vi "FF_WriteAnkleTraj.vi"(8 "error in (no error)":errorcluster, 10 "AnkleTraj":T1(array[cluster]), 11 "ForceField in":refnum<class "ForceField.lvclass">) -> (0 "error out":errorcluster, 3 "ForceField out":refnum<class "ForceField.lvclass">)   [LabVIEW 2015, in "ForceField.lvclass"]
uses:
  ForceField.lvclass
  ForceField.lvclass/ForceField.ctl
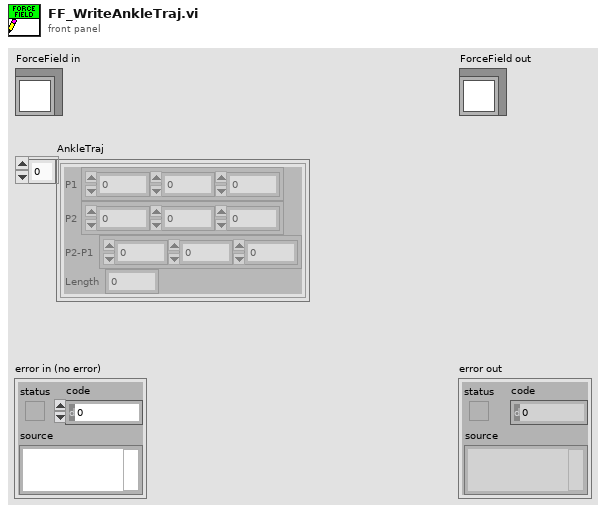
[diagram p1: front panel]
types:
  T1 = cluster{"P1":dbl[], "P2":dbl[], "P2-P1":dbl[], "Length":dbl}[]
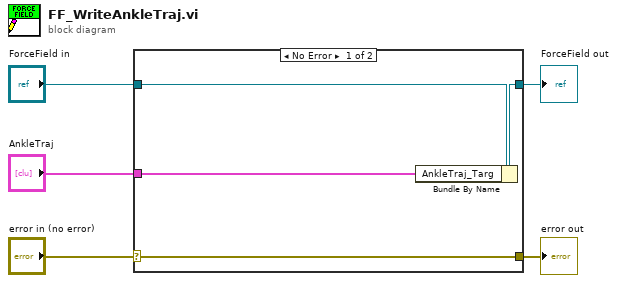
[diagram p0: block diagram]
diagram:
  n1 = case shown="No Error" "error in (no error)" {
    selector: "error in (no error)" -> [w9 w10]
    tunnel: [w9 w10] -> w4
    tunnel: [w7 w11] -> w2
    tunnel: "ForceField in" -> [w8 w11]
    tunnel: "AnkleTraj" -> [w6 _]
    frame No Error {
      n2 = Bundle By Name(cluster=w8, "AnkleTraj_Targ"=w6) -> (w7:refnum<class "ForceField.lvclass">)
    }
    frame Error {
    }
  }
  "error out" <- w4
  "ForceField out" <- w2
